vi "alarm clock - fancy.vi"(7 "action":enum16{"init", "check", "start", "stop"}(ring), 8 "alarm":T1={"counter (min)"=1600.0, "alarm"=FALSE, "start"=TRUE, "set (min)"=1600.0, "stop"=TRUE} {"set (min)" format="%_4f"; "counter (min)" format="%_4f"}, 11 "seconds":i32) -> (0 "alarm out":T1={"counter (min)"=1600.0, "alarm"=FALSE, "start"=TRUE, "set (min)"=1600.0, "stop"=TRUE} {"set (min)" format="%_4f"; "counter (min)" format="%_4f"}, 3 "alarm!":bool)   [LabVIEW 2015]
uses:
  alarm clock control.ctl
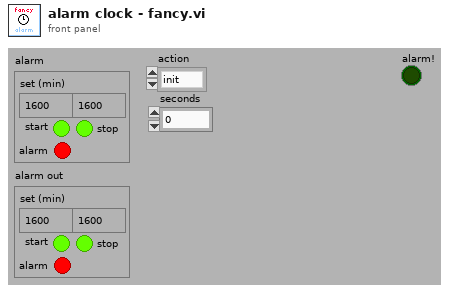
[diagram p1: front panel]
types:
  T1 = typedef "alarm clock control.ctl" = cluster{"counter (min)":dbl, "alarm":bool, "start":bool, "set (min)":dbl, "stop":bool}
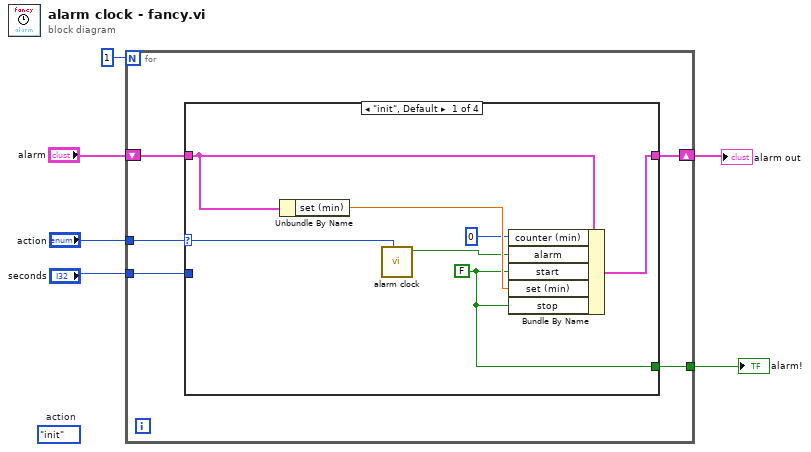
[diagram p0: block diagram]
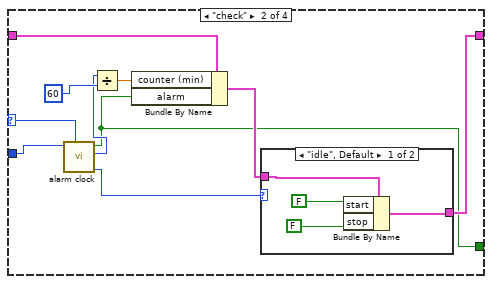
[diagram p2: hidden frame]
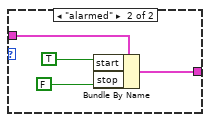
[diagram p3: hidden frame]
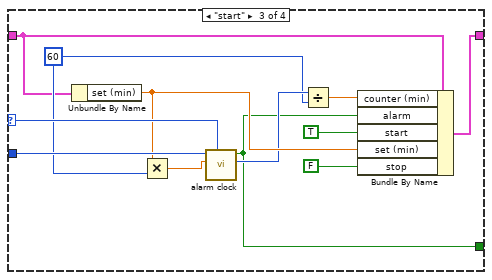
[diagram p4: hidden frame]
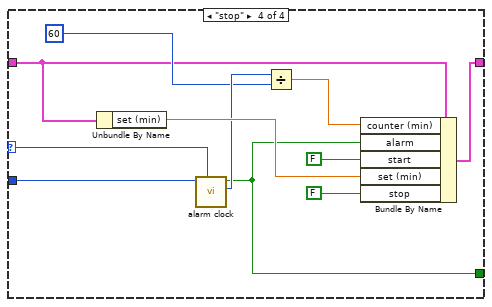
[diagram p5: hidden frame]
diagram:
  (unwired) enum16{"init", "check", "start", "stop"}."init"  # action
  n1 = for {
    N: u32 1 ("milliseconds per cycle") -> [_]
    shift-right: [w10] -> w5
    shift-left: "alarm" -> [w11]
    tunnel: "action" -> [w9]
    tunnel: "seconds" -> [w8]
    tunnel: [w7] -> w1
    n2 = case shown="\"init\", Default" w9 {
      selector: w9 -> [w14 w25 w47 w51]
      tunnel: w11 -> [w16 w28 w38 w52]
      tunnel: [w15 w21 w39 w53] -> w10
      tunnel: w8 -> [_ w24 w48 w50]
      tunnel: [w13 w19 w37 w49] -> w7
      frame "init", Default {
        w13 = FALSE
        n3 = Unbundle By Name(w16) -> ("set (min)"=w18:dbl)
        n4 = call "alarm clock.vi"("action"=w14) -> ("alarm"=w12:bool)  [unwired: 8 in, 2 out]
        n5 = Bundle By Name(cluster=w16, "counter (min)"=u32 0 ("milliseconds per cycle"), "alarm"=w12, "start"=w13, "set (min)"=w18, "stop"=w13) -> (w15:T1)
      }
      frame "check" {
        n6 = call "alarm clock.vi"("action"=w25, "seconds"=w24) -> ("state"=w22:enum16{"idle", "alarmed"}, "tics"=w23:i32, "alarm"=w19:bool)  [unwired: 7 in]
        n7 = Divide(x=w23, y=u32 60 ("milliseconds per cycle")) -> (x/y=w26:dbl)
        n8 = Bundle By Name(cluster=w28, "counter (min)"=w26, "alarm"=w19) -> (w20:T1)
        n9 = case shown="\"idle\", Default" w22 {
          tunnel: [w30 w36] -> w21
          tunnel: w20 -> [w29 w35]
          frame "idle", Default {
            n10 = Bundle By Name(cluster=w29, "start"=FALSE, "stop"=FALSE) -> (w30:T1)
          }
          frame "alarmed" {
            n11 = Bundle By Name(cluster=w35, "start"=TRUE, "stop"=FALSE) -> (w36:T1)
          }
        }
      }
      frame "start" {
        w41 = u32 60 ("milliseconds per cycle")
        n12 = Unbundle By Name(w38) -> ("set (min)"=w46:dbl)
        n13 = Multiply(x=w46, y=w41) -> (x*y=w45:dbl)
        n14 = call "alarm clock.vi"("action"=w47, "alarm time"=w45, "seconds"=w48) -> ("tics"=w42:i32, "alarm"=w37:bool)  [unwired: 6 in, 1 out]
        n15 = Divide(x=w42, y=w41) -> (x/y=w40:dbl)
        n16 = Bundle By Name(cluster=w38, "counter (min)"=w40, "alarm"=w37, "start"=TRUE, "set (min)"=w46, "stop"=FALSE) -> (w39:T1)
      }
      frame "stop" {
        n17 = Unbundle By Name(w52) -> ("set (min)"=w59:dbl)
        n18 = call "alarm clock.vi"("action"=w51, "seconds"=w50) -> ("tics"=w56:i32, "alarm"=w49:bool)  [unwired: 7 in, 1 out]
        n19 = Divide(x=w56, y=u32 60 ("milliseconds per cycle")) -> (x/y=w54:dbl)
        n20 = Bundle By Name(cluster=w52, "counter (min)"=w54, "alarm"=w49, "start"=FALSE, "set (min)"=w59, "stop"=FALSE) -> (w53:T1)
      }
    }
  }
  "alarm out" <- w5
  "alarm!" <- w1
